vi "Limited Integrator (DBL Array).vi"(4 "initialize":bool, 6 "bounds":cluster{"upper bound":dbl, "lower bound":dbl}[](array[cluster]) {"lower bound" format="%.2f"; "upper bound" format="%.2f"}, 7 "dt":dbl=1e-09 min=1e-09 format="%.6f", 9 "initial conditions":dbl[](array[numeric]) format="%.2f", 10 "input points":dbl[](array[numeric]) format="%.2f") -> (3 "output points":dbl[](array[numeric]) format="%.2f")   [LabVIEW 2017, in "NI_AdvCtrl_continuous linear.lvlib"]
doc: "LabVIEW no longer supports this VI. You can obtain similar functionality by installing the LabVIEW Simulation Module.\n\nIntegrates a continuous input signal where limits are given. The integration process is based on Euler method. dt must be positive. The result of the integration process is in between of lower bound and upper bound."
uses:
  <vilib>/addons/control/advanced/NI_AdvCtrl_continuous linear.lvlib
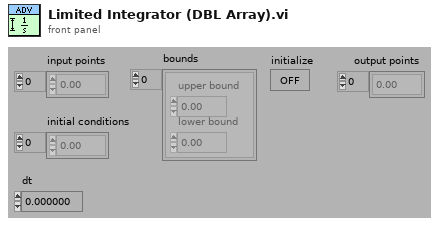
[diagram p1: front panel]
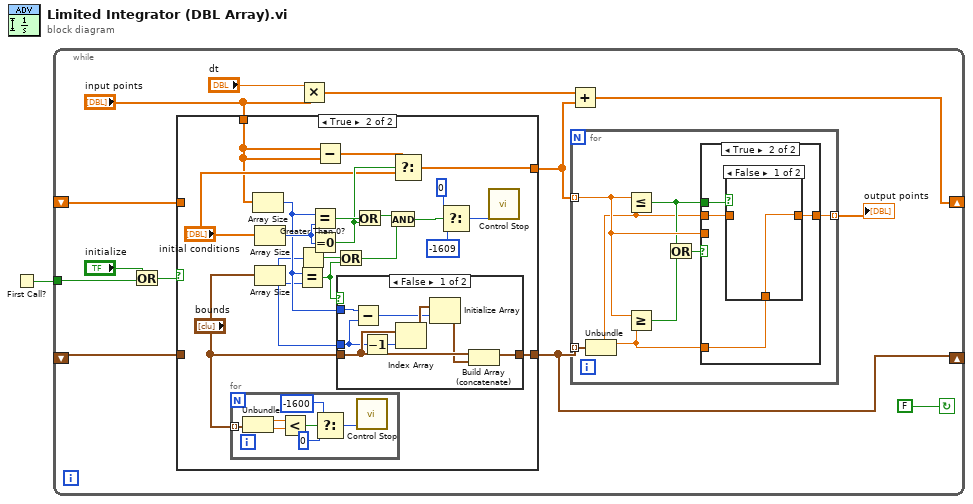
[diagram p0: block diagram]
diagram:
  n1 = First Call?() -> (First Call?: T/F=w1:bool)
  n2 = while {
    shift-left: _ -> [w7]
    shift-right: [w8] -> _
    tunnel: w1 -> [w10]
    shift-left: _ -> [w11]
    shift-right: [w2] -> _
    stop <- FALSE continue-if-true
    n3 = Or(x="initialize", y=w10) -> (x .or. y?=w12:bool)
    n4 = case shown="True" w12 {
      tunnel: "input points" -> [_ w18]
      tunnel: [w15 w30] -> w3
      tunnel: w11 -> [w15 _]
      tunnel: [w16 w28] -> w8
      tunnel: w7 -> [w16 _]
      frame False {
      }
      frame True {
        n5 = for {
          tunnel: "bounds" -> [w42] mode=indexing
          n6 = Unbundle(w42) -> ("upper bound"=w41:dbl, "lower bound"=w40:dbl)
          n7 = Less?(x=w41, y=w40) -> (x < y?=w39:bool)
          n8 = Select(t=-1600, s=w39, f=0) -> (s? t:f=w38:i32)
          n9 = call <vilib>:"Control Stop.vi"("error"=w38) -> ()  [unwired: 2 out]
        }
        n10 = Array Size(array=w18) -> (size(s)=w29:i32)
        n11 = Array Size(array="initial conditions") -> (size(s)=w33:i32)
        n12 = Array Size(array="bounds") -> (size(s)=w23:i32)
        n13 = Equal?(x=w29, y=w23) -> (x = y?=w24:bool)
        n14 = Greater Than 0?(x=w23) -> (x > 0?=w22:bool)
        n15 = Equal?(x=w29, y=w33) -> (x = y?=w31:bool)
        n16 = Equal To 0?(x=w33) -> (x = 0?=w25:bool)
        n17 = Subtract(x=w18, y=w18) -> (x-y=w17:dbl[])
        n18 = Or(x=w22, y=w24) -> (x .or. y?=w21:bool)
        n19 = case shown="False" w24 {
          tunnel: [w50 w51] -> w28
          tunnel: "bounds" -> [w49 w51]
          tunnel: w23 -> [w44 _]
          tunnel: w29 -> [w45 _]
          frame False {
            n20 = Subtract(x=w45, y=w44) -> (x-y=w43:i32)
            n21 = Decrement(x=w44) -> (x-1=w48:i32)
            n22 = Index Array(array=w49, index=w48) -> (element=w47:cluster{"upper bound":dbl, "lower bound":dbl})
            n23 = Initialize Array(w47, w43) -> (w46:cluster{"upper bound":dbl, "lower bound":dbl}[])
            n24 = Build Array (concatenate)(w49, w46) -> (w50:cluster{"upper bound":dbl, "lower bound":dbl}[])
          }
          frame True {
          }
        }
        n25 = Or(x=w31, y=w25) -> (x .or. y?=w32:bool)
        n26 = And(x=w32, y=w21) -> (x .and. y?=w26:bool)
        n27 = Select(t=w17, s=w25, f="initial conditions") -> (s? t:f=w30:dbl[])
        n28 = Select(t=0, s=w26, f=-1609) -> (s? t:f=w20:i32)
        n29 = call <vilib>:"Control Stop.vi"("error"=w20) -> ()  [unwired: 2 out]
      }
    }
    n30 = Multiply(x="dt", y="input points") -> (x*y=w4:dbl[])
    n31 = Add(x=w4, y=w3) -> (x+y=w2:dbl[])
    n32 = for {
      tunnel: [w58] -> w14 mode=indexing
      tunnel: w3 -> [w57] mode=indexing
      tunnel: w8 -> [w54] mode=indexing
      n33 = Unbundle(w54) -> ("upper bound"=w52:dbl, "lower bound"=w53:dbl)
      n34 = Less Or Equal?(x=w57, y=w53) -> (x <= y?=w56:bool)
      n35 = Greater Or Equal?(x=w57, y=w52) -> (x >= y?=w55:bool)
      n36 = Or(x=w56, y=w55) -> (x .or. y?=w59:bool)
      n37 = case shown="True" w59 {
        tunnel: [w60 w62] -> w58
        tunnel: w57 -> [w60 _]
        tunnel: w56 -> [_ w64]
        tunnel: w53 -> [_ w63]
        tunnel: w52 -> [_ w61]
        frame False {
        }
        frame True {
          n38 = case shown="False" w64 {
            tunnel: w63 -> [_ w66]
            tunnel: [w65 w66] -> w62
            tunnel: w61 -> [w65 _]
            frame False {
            }
            frame True {
            }
          }
        }
      }
    }
    "output points" <- w14
  }
